vi "Outputs.vi"(11 "OutputsCluster":T1) -> ()   [LabVIEW 2012]
uses:
  Outputs_All.ctl
  Flywheel/Outputs_Flywheel.ctl
  tankdrive/Output_Wheel_Speeds.ctl
  Conveyor/Conveyor_outputs.ctl
  Conveyor/Conveyor module state.ctl
  Conveyor/Conveyor_outputsV2.ctl
  Conveyor/3-Ball-Conveyor_Module_State.ctl
  Conveyor/T_Roller module state.ctl
  Turret/Outputs_Turret.ctl
  Roller/Outputs_Roller.ctl
  Bridge Tipper/Outputs_Tipper.ctl
panel:
  out "error out":errorcluster
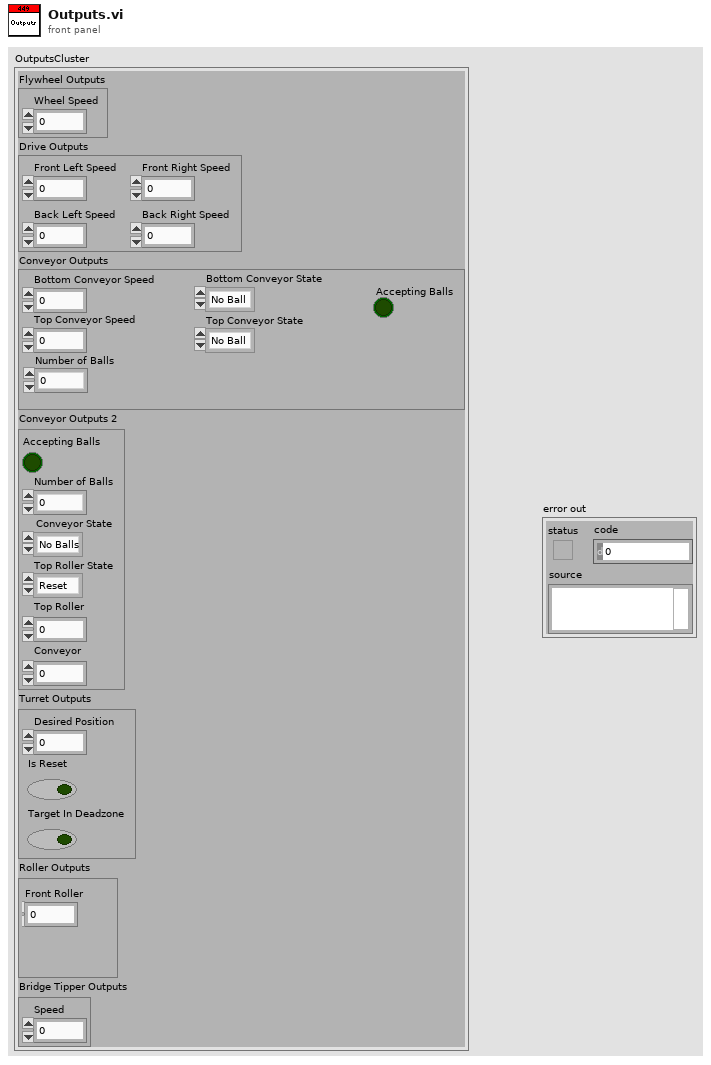
[diagram p1: front panel]
types:
  T1 = typedef "Outputs_All.ctl" = cluster{"Flywheel Outputs":T2, "Drive Outputs":T3, "Conveyor Outputs":T4, "Conveyor Outputs 2":T6, "Turret Outputs":T9, "Roller Outputs":T10, "Bridge Tipper Outputs":T11}
  T2 = typedef "Outputs_Flywheel.ctl" = cluster{"Wheel Speed":dbl}
  T3 = typedef "Output_Wheel_Speeds.ctl" = cluster{"Front Left Speed":dbl, "Front Right Speed":dbl, "Back Left Speed":dbl, "Back Right Speed":dbl}
  T4 = typedef "Conveyor_outputs.ctl" = cluster{"Bottom Conveyor Speed":dbl, "Top Conveyor Speed":dbl, "Bottom Conveyor State":T5, "Top Conveyor State":T5, "Accepting Balls":bool, "Number of Balls":i32}
  T5 = typedef "Conveyor module state.ctl" = enum16{"No Ball", "Has Ball", "Ball Below Hold", "Ball Above Hold", "Outputting Ball", "Reset"}
  T6 = typedef "Conveyor_outputsV2.ctl" = cluster{"Accepting Balls":bool, "Number of Balls":i32, "Conveyor State":T7, "Top Roller State":T8, "Top Roller":dbl, "Conveyor":dbl}
  T7 = typedef "3-Ball-Conveyor_Module_State.ctl" = enum16{"No Balls", "Collecting Ball", "Holding 1", "Pushing Ball Out", "Holding 2", "Lowering Ball", "Reset", "Disabled"}
  T8 = typedef "T_Roller module state.ctl" = enum16{"Reset", "Disabled", "Waiting for Ball", "Holding", "Ball not far enough", "Ball too far", "Firing"}
  T9 = typedef "Outputs_Turret.ctl" = cluster{"Desired Position":dbl, "Is Reset":bool, "Target In Deadzone":bool}
  T10 = typedef "Outputs_Roller.ctl" = cluster{"Front Roller":dbl}
  T11 = typedef "Outputs_Tipper.ctl" = cluster{"Speed":dbl}
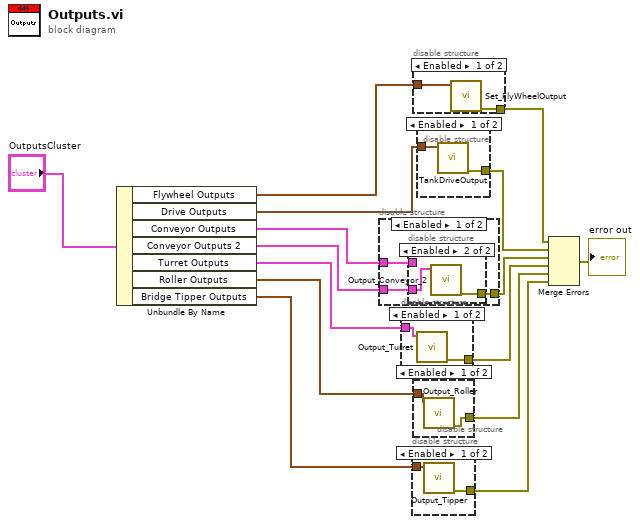
[diagram p0: block diagram]
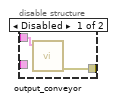
[diagram p3: hidden frame]
diagram:
  n1 = Unbundle By Name("OutputsCluster") -> ("Flywheel Outputs"=w14:T2, "Drive Outputs"=w13:T3, "Conveyor Outputs"=w12:T4, "Conveyor Outputs 2"=w1:T6, "Turret Outputs"=w2:T9, "Roller Outputs"=w11:T10, "Bridge Tipper Outputs"=w4:T11)
  n2 = disable-structure shown="Enabled" {
    disable-tunnel: w12 -> [w18 _]
    disable-tunnel: [w17 _] -> w8
    disable-tunnel: w1 -> [w16 _]
    frame Enabled {
      n3 = disable-structure shown="Enabled" {
        disable-tunnel: w18 -> [w20 _]
        disable-tunnel: [w19 w22] -> w17
        disable-tunnel: w16 -> [_ w21]
        frame Disabled {
          n4 = call "output_conveyor.vi"("Conveyor_outputs"=w20) -> ("error out"=w19:errorcluster)  [unwired: 10 in]
        }
        frame Enabled {
          n5 = call "Output_Conveyor_2.vi"("Conveyor Outputs in"=w21) -> ("error out"=w22:errorcluster)  [unwired: 10 in]
        }
      }
    }
    frame Disabled {
    }
  }
  n6 = disable-structure shown="Enabled" {
    disable-tunnel: w2 -> [w24 _]
    disable-tunnel: [w23 _] -> w7
    frame Enabled {
      n7 = call "Output_Turret.vi"("Turret Outputs"=w24) -> ("error out"=w23:errorcluster)  [unwired: 10 in]
    }
    frame Disabled {
    }
  }
  n8 = disable-structure shown="Enabled" {
    disable-tunnel: w4 -> [w26 _]
    disable-tunnel: [w25 _] -> w3
    frame Enabled {
      n9 = call "Output_Tipper.vi"("Bridge Tipper Outputs"=w26) -> ("error out"=w25:errorcluster)  [unwired: 10 in]
    }
    frame Disabled {
    }
  }
  n10 = disable-structure shown="Enabled" {
    disable-tunnel: w14 -> [w28 _]
    disable-tunnel: [w27 _] -> w10
    frame Enabled {
      n11 = call "Set_FlyWheelOutput.vi"("FlyWheelOutputs"=w28) -> ("error out"=w27:errorcluster)  [unwired: 10 in]
    }
    frame Disabled {
    }
  }
  n12 = disable-structure shown="Enabled" {
    disable-tunnel: w11 -> [w30 _]
    disable-tunnel: [w29 _] -> w6
    frame Enabled {
      n13 = call "Output_Roller.vi"("Roller Outputs"=w30) -> ("error out"=w29:errorcluster)  [unwired: 10 in]
    }
    frame Disabled {
    }
  }
  n14 = disable-structure shown="Enabled" {
    disable-tunnel: w13 -> [w32 _]
    disable-tunnel: [w31 _] -> w9
    frame Enabled {
      n15 = call "TankDriveOutput.vi"("Drive Outputs"=w32) -> ("error out"=w31:errorcluster)  [unwired: 10 in]
    }
    frame Disabled {
    }
  }
  n16 = Merge Errors(w10, w9, w8, w7, w6, w3) -> (→"error out":errorcluster)
